vi "Draw Wings.vi"(9 "draw options":T1={"Text Color"=16777238, "Wing Color"=16751616, "Dial Outline Color"=13816530, "Sky Color"=3381759, "Ground Color"=8213043, "Horizon Line Color"=16777225, "Outline Color"=0, "Dial Background Color"=5987163, "Draw Wings"=TRUE, "Draw Text"=TRUE, "Font Name"="Helvetica", "Angle units"=enum."Degrees"}, 10 "draw area state":T3, 11 "picture in":picture) -> (3 "picture out":picture)   [LabVIEW 2017, in "NI_Robotics_Attitude Picture.lvlib"]
uses:
  <vilib>/robotics/Controls/Attitude Indicator/Attitude Picture/NI_Robotics_Attitude Picture.lvlib
  <vilib>/robotics/Controls/Attitude Indicator/Attitude Picture/Draw Area State.ctl
  <vilib>/Utility/miscctls.llb/LVBoundsTypeDef.ctl
  <vilib>/robotics/Controls/Attitude Indicator/Attitude Picture/Draw Options.ctl
  <vilib>/robotics/Controls/Utilities/Angle Units.ctl
  <vilib>/Analysis/coordinate.llb/2D Cartesian Coordinate Rotation.vi
  <vilib>/Analysis/coordinate.llb/2D Cartesian Coordinate Rotation (Array).vi
  <vilib>/robotics/Controls/Utilities/NI_Robotics_Control Utilities.lvlib
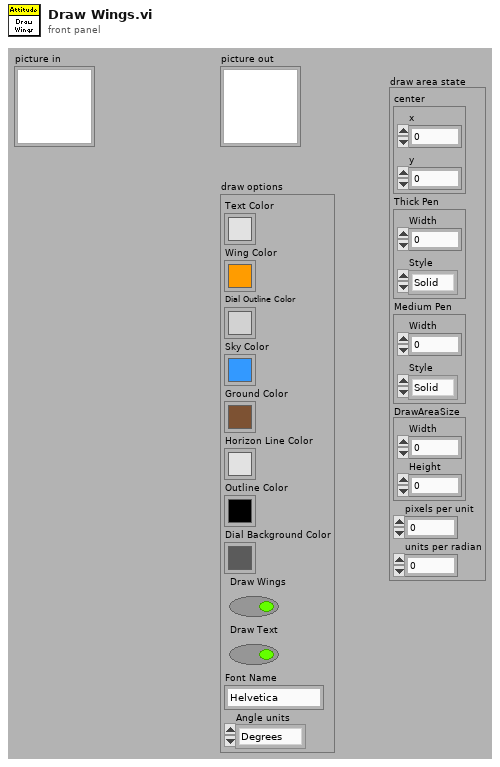
[diagram p1: front panel]
types:
  T1 = typedef "NI_Robotics_Attitude Picture.lvlib/Draw Options.ctl" = cluster{"Text Color":u32, "Wing Color":u32, "Dial Outline Color":u32, "Sky Color":u32, "Ground Color":u32, "Horizon Line Color":u32, "Outline Color":u32, "Dial Background Color":u32, "Draw Wings":bool, "Draw Text":bool, "Font Name":string, "Angle units":T2}
  T2 = typedef "NI_Robotics_Control Utilities.lvlib/Angle Units.ctl" = enum16{"Radians", "Degrees"}
  T3 = typedef "NI_Robotics_Attitude Picture.lvlib/Draw Area State.ctl" = cluster{"center":cluster{"x":i16, "y":i16}, "Thick Pen":cluster{"Width":u16, "Style":enum32{"Solid", "Dash", "Dot", "DashDot", "DashDotDot"}}, "Medium Pen":cluster{"Width":u16, "Style":enum32{"Solid", "Dash", "Dot", "DashDot", "DashDotDot"}}, "DrawAreaSize":T4, "pixels per unit":dbl, "units per radian":dbl}
  T4 = typedef "LVBoundsTypeDef.ctl" = cluster{"Width":u32, "Height":u32}
  T5 = cluster{"Width":u16, "Style":enum32{"Solid", "Dash", "Dot", "DashDot", "DashDotDot"}}
  T6 = cluster{"Width":u16, "Style":enum32{"Solid", "Dash", "Dot", "DashDot", "DashDotDot"}}[]
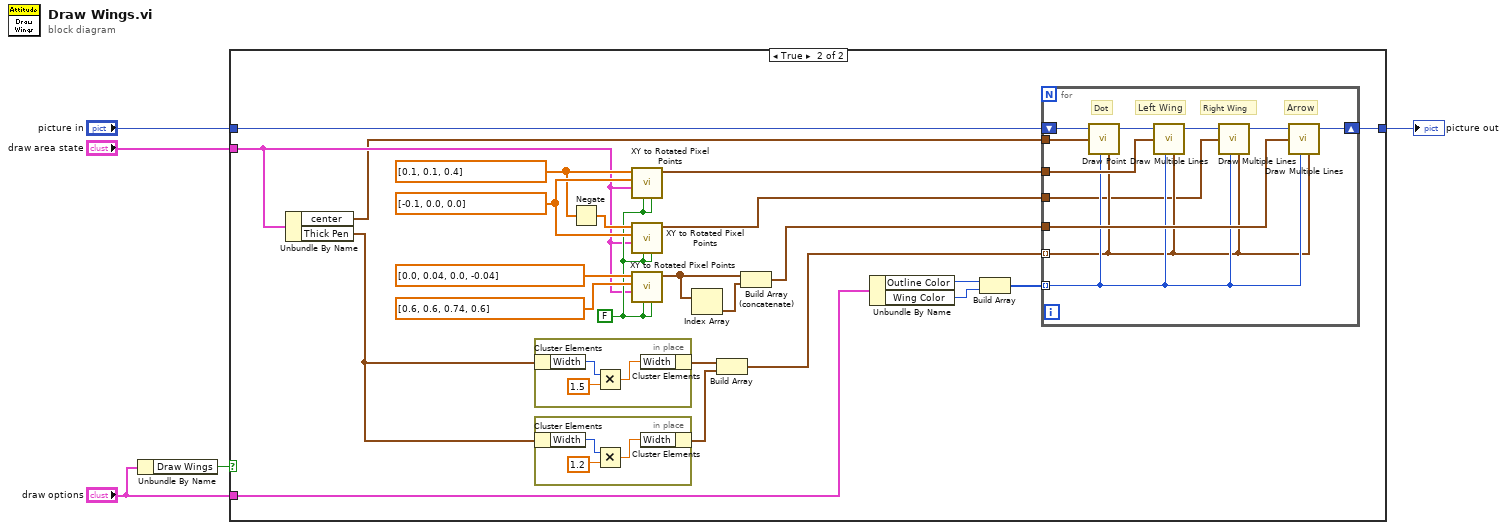
[diagram p0: block diagram]
diagram:
  n1 = Unbundle By Name("draw options") -> ("Draw Wings"=w1:bool)
  n2 = case shown="True" w1 {
    tunnel: "picture in" -> [w6 w28]
    tunnel: [w6 w26] -> w4
    tunnel: "draw area state" -> [_ w12]
    tunnel: "draw options" -> [_ w23]
    frame False {
    }
    frame True {
      w16 = dbl[] [-0.1, 0.0, 0.0]
      w15 = dbl[] [0.1, 0.1, 0.4]
      w13 = FALSE ("use pitch")
      n3 = Unbundle By Name(w12) -> ("center"=w11:cluster{"x":i16, "y":i16}, "Thick Pen"=w8:T5)
      n4 = in-place {
        n5 = in-place-cluster #1(w8) -> ("Width"=w35:u16)
        n6 = Multiply(x=w35, y=1.5) -> (x*y=w33:dbl)
        n7 = in-place-cluster #1("Width"=w33) -> (w22:T5)
      }
      n8 = in-place {
        n9 = in-place-cluster #2(w8) -> ("Width"=w32:u16)
        n10 = Multiply(x=w32, y=1.2) -> (x*y=w30:dbl)
        n11 = in-place-cluster #2("Width"=w30) -> (w7:T5)
      }
      n12 = Negate(x=w15) -> (-x=w14:dbl[])
      n13 = call <vilib>:"XY to Rotated Pixel Points.vi"("use roll"=w13, "use pitch"=w13, "draw area state"=w12, "unrotated y (units)"=w16, "unrotated x (units)"=w15) -> ("rotated pixel points"=w10:cluster{"x":i16, "y":i16}[])  [unwired: 6 in]
      n14 = call <vilib>:"XY to Rotated Pixel Points.vi"("use roll"=w13, "use pitch"=w13, "draw area state"=w12, "unrotated y (units)"=w16, "unrotated x (units)"=w14) -> ("rotated pixel points"=w9:cluster{"x":i16, "y":i16}[])  [unwired: 6 in]
      n15 = call <vilib>:"XY to Rotated Pixel Points.vi"("use roll"=w13, "use pitch"=w13, "draw area state"=w12, "unrotated y (units)"=dbl[] [0.6, 0.6, 0.74, 0.6], "unrotated x (units)"=dbl[] [0.0, 0.04, 0.0, -0.04]) -> ("rotated pixel points"=w19:cluster{"x":i16, "y":i16}[])  [unwired: 6 in]
      n16 = Index Array(array=w19) -> (element=w20:cluster{"x":i16, "y":i16})  [unwired: 1 in]
      n17 = Build Array(w22, w7) -> (w27:T6)
      n18 = Build Array (concatenate)(w19, w20) -> (w18:cluster{"x":i16, "y":i16}[])
      n19 = Unbundle By Name(w23) -> ("Outline Color"=w25:u32, "Wing Color"=w24:u32)
      n20 = Build Array(w25, w24) -> (w29:u32[])
      n21 = for {
        tunnel: w29 -> [w39] mode=indexing
        tunnel: w27 -> [w38] mode=indexing
        shift-right: [w45] -> w26
        shift-left: w28 -> [w43]
        tunnel: w18 -> [w46]
        tunnel: w11 -> [w44]
        tunnel: w10 -> [w41]
        tunnel: w9 -> [w37]
        # "Arrow"
        # "Right Wing"
        # "Left Wing"
        # "Dot"
        n22 = call <vilib>:"Draw Point.vi"("picture"=w43, "point(x,y)"=w44, "color(black)"=w39, "pen"=w38) -> ("new picture"=w42:picture)  [unwired: 5 in]
        n23 = call <vilib>:"Draw Multiple Lines.vi"("picture"=w42, "line endpoints"=w41, "color(black)"=w39, "pen"=w38) -> ("new picture"=w40:picture)  [unwired: 5 in]
        n24 = call <vilib>:"Draw Multiple Lines.vi"("picture"=w40, "line endpoints"=w37, "color(black)"=w39, "pen"=w38) -> ("new picture"=w36:picture)  [unwired: 5 in]
        n25 = call <vilib>:"Draw Multiple Lines.vi"("picture"=w36, "line endpoints"=w46, "color(black)"=w39, "pen"=w38) -> ("new picture"=w45:picture)  [unwired: 5 in]
      }
    }
  }
  "picture out" <- w4
